vi "Read HW Torque 5.vi"(6 "error in":errorcluster, 8 "MaxRead":i32, 9 "Channel in":u16) -> (0 "error out":errorcluster, 1 "Messages":T1(array[cluster]), 2 "Pass":bool, 3 "Channel out":u16)   [LabVIEW 2023]
uses:
  7ad73885-74d4-4865-958d-ac69876d8a76.vi
  Communication/PCAN2023/PCAN API.lvlib
panel:
  out "reversed array":u8[](array[numeric]) format="%.0x"
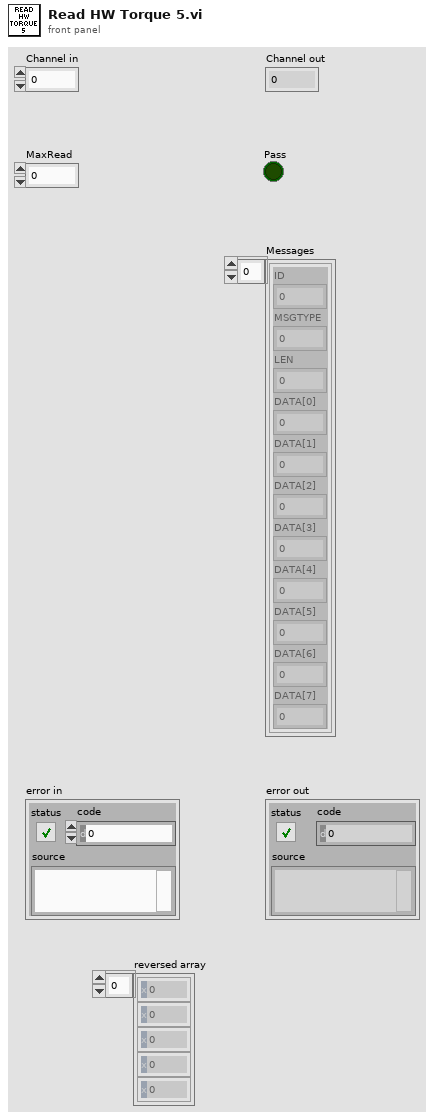
[diagram p1: front panel]
types:
  T1 = cluster{"ID":u32, "MSGTYPE":u8, "LEN":u8, "DATA[0]":u8, "DATA[1]":u8, "DATA[2]":u8, "DATA[3]":u8, "DATA[4]":u8, "DATA[5]":u8, "DATA[6]":u8, "DATA[7]":u8}[]
  T2 = cluster{"ID":u32, "MSGTYPE":u8, "LEN":u8, "DATA[0]":u8, "DATA[1]":u8, "DATA[2]":u8, "DATA[3]":u8, "DATA[4]":u8, "DATA[5]":u8, "DATA[6]":u8, "DATA[7]":u8}
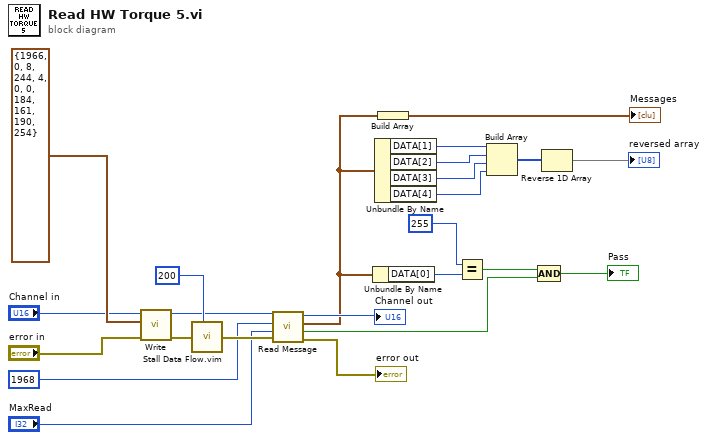
[diagram p0: block diagram]
diagram:
  n1 = call "Write.vi"("error in"="error in", "MessageBuffer"=T2 {"ID"=1966, "MSGTYPE"=0, "LEN"=8, "DATA[0]"=244, "DATA[1]"=4, "DATA[2]"=0, "DATA[3]"=0, "DATA[4]"=184, "DATA[5]"=161, "DATA[6]"=190, "DATA[7]"=254}, "Channel"="Channel in") -> ("error out"=w23:errorcluster, "Channel out"=w8:u16)  [unwired: 5 in, 2 out]
  n2 = call "Stall Data Flow.vim"("value in"=w23, "milliseconds to wait"=u32 200) -> ("value out"=w7:errorcluster)  [unwired: 1 out]
  n3 = call "Read Message.vi"("error in"=w7, "MaxRead"="MaxRead", "ID"=u32 1968, "Channel in"=w8) -> ("error out"=→"error out":errorcluster, "Passed"=w1:bool, "Last Message"=w2:T2, "Channel out"=→"Channel out":u16)  [unwired: 3 in, 1 out]
  n4 = Unbundle By Name(w2) -> ("DATA[0]"=w20:u8)
  n5 = Unbundle By Name(w2) -> ("DATA[1]"=w16:u8, "DATA[2]"=w15:u8, "DATA[3]"=w14:u8, "DATA[4]"=w13:u8)
  n6 = Build Array(w2) -> (→"Messages":T1)
  n7 = Equal?(x=u8 255, y=w20) -> (x = y?=w18:bool)
  n8 = Build Array(w16, w15, w14, w13) -> (w12:u8[])
  n9 = Compound Arithmetic op=AND(w18, w1) -> (→"Pass":bool)
  n10 = Reverse 1D Array(array=w12) -> (reversed array=→"reversed array":u8[])
